vi "grabber stim laser control panel.vi"() -> ()   [LabVIEW 2010]
uses:
  FPGA_ref.ctl
  <vilib>/Platform/TimedLoop/XDataNode/XDataNode.xnode
  <vilib>/Platform/TimedLoop/XDataNode/timing_clust.ctl
  <vilib>/Platform/TimedLoop/XDataNode/nitl_modes.ctl
  <vilib>/Platform/TimedLoop/XDataNode/wakeup.ctl
  <vilib>/rvi/interface/nirviReadWriteControl/nirviReadWriteControl.xnode
  <vilib>/rvi/interface/common/niFpgaNodeNameForErrorReporting.ctl
  <vilib>/rvi/errors/niLvFpgaWhatHappensToTopLevelVI.ctl
  <vilib>/Utility/error.llb/Error Cluster From Error Code.vi
  <vilib>/rvi/errors/niLvFpgaAdjustHostInterfaceError.vi
  <vilib>/Platform/TimedLoop/XDataNode/XDNodeRunTimeDep.lvlib
  NiFpgaLv.dll
panel:
  in  "FPGARef":T1
  in  "laser ref":refnum<vi>
  out "time since last stim":u32
  in  "stop":bool
  in  "auto trig":bool
  in  "stim period (s)":dbl format="%#_3p"
  in  "stim duration (s)":dbl format="%#_3p"
  in  "stim laser on":bool
  # "set to <= 0 for full manual control"
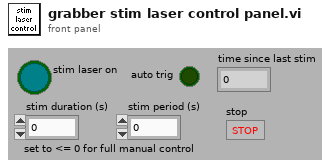
[diagram p1: front panel]
types:
  T1 = typedef "FPGA_ref.ctl" = refnum<k20>
  T2 = typedef "XDNodeRunTimeDep.lvlib/timing_clust.ctl" = cluster{"Expected End [f-1]":u64, "Actual End [f-1]":u64, "Finished Late? [f-1]":bool, "Expected End [i-1]":u64, "Actual End [i-1]":u64, "Finished Late? [i-1]":bool, "Expected Start [i]":u64, "Actual Start [i]":u64, "Expected Start [f]":u64, "Actual Start [f]":u64, "Source Name":string, "Structure Name":string, "Period":i64, "Deadline":i64, "Offset":i64, "Start":i64, "Priority":i32, "Timeout":i32, "Mode":T3, "Wakeup Reason":T4, "Error":errorcluster, "Source Type":string, "Secondary Source Type":string, "Global End Time":u64, "Global Start Time":u64, "Frame Duration":u64, "Iteration Duration":u64, "Assigned CPU":i32, "I/O Scan Engine Mode":u32}
  T3 = typedef "XDNodeRunTimeDep.lvlib/nitl_modes.ctl" = enum32{"No Change", "Process missed periods, maintain original phase", "Discard missed periods, maintain original phase", "Process missed periods, ignore original phase", "Discard missed periods, ignore original phase"}
  T4 = typedef "XDNodeRunTimeDep.lvlib/wakeup.ctl" = enum32{"Normal", "Aborted", "Asynchronous wakeup", "Timing source error", "Timed loop error", "Timeout"}
  T5 = typedef "niFpgaNodeNameForErrorReporting.ctl" = enum16{"Open FPGA VI Reference", "Read/Write Control", "Invoke Method: Abort", "Invoke Method: Acknowledge IRQ", "Invoke Method: Download", "Invoke Method: FIFO.Configure", "Invoke Method: FIFO.Read", "Invoke Method: FIFO.Start", "Invoke Method: FIFO.Stop", "Invoke Method: FIFO.Write", "Invoke Method: Reset", "Invoke Method: Run", "Invoke Method: Wait on IRQ", "Close FPGA VI Reference"}
  T6 = typedef "niLvFpgaWhatHappensToTopLevelVI.ctl" = enum16{"top level VI scripted behind XNode", "top level VI inlined behind XNode"}
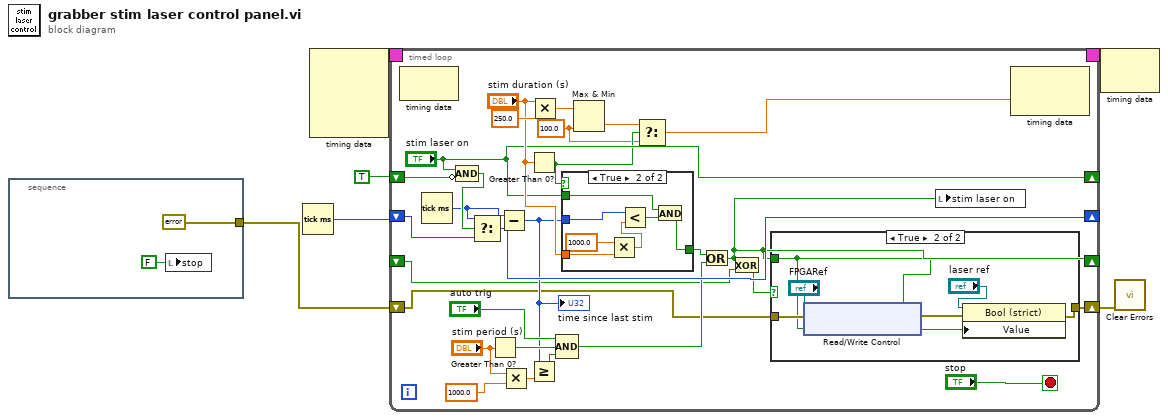
[diagram p0: block diagram]
diagram:
  n1 = stacked-sequence {
    tunnel: [errorcluster {"status"=FALSE, "code"=0, "source"=""} ("error out")] -> w1
    frame #0 {
      n2 = local write "stop"(FALSE ("stop")) -> ()
    }
  }
  n3 = Tick Count (ms)() -> (millisecond timer value=w4:u32)
  n4 = node-c288() -> (w6:T2)  [unwired: 4 in]
  n5 = timed-loop {
    timing: w6 -> [_]
    timing-out: [_] -> w5
    shift-right: ["stim laser on"] -> _
    shift-left: TRUE ("stim laser on") -> [w33]
    shift-right: [w27] -> _
    shift-left: w4 -> [w31]
    shift-right: [w13] -> w2
    shift-left: w1 -> [w12]
    shift-right: [w11] -> _
    shift-left: _ -> [w10]
    stop <- "stop" stop-if-true
    w15 = 100.0 ("y")
    n6 = node-c288() -> ()  [unwired: 1 in, 1 out]
    n7 = Tick Count (ms)() -> (millisecond timer value=w21:u32)
    n8 = Compound Arithmetic op=AND("stim laser on", invert w33) -> (w32:bool)
    n9 = Select(t=w21, s=w32, f=w31) -> (s? t:f=w27:u32)
    n10 = Greater Than 0?(x="stim period (s)") -> (x > 0?=w29:bool)
    n11 = Subtract(x=w21, y=w27) -> (x-y=w23:u32)
    "time since last stim" <- w23
    n12 = Multiply(x="stim period (s)", y=1000.0 ("x")) -> (x*y=w24:dbl)
    n13 = Greater Than 0?(x="stim duration (s)") -> (x > 0?=w17:bool)
    n14 = Greater Or Equal?(x=w23, y=w24) -> (x >= y?=w22:bool)
    n15 = Multiply(x="stim duration (s)", y=250.0) -> (x*y=w34:dbl)
    n16 = Compound Arithmetic op=AND("auto trig", w29, w22) -> (w20:bool)
    n17 = case shown="True" w17 {
      tunnel: "stim duration (s)" -> [_ w90]
      tunnel: [w83 w85] -> w19
      tunnel: "stim laser on" -> [w83 w84]
      tunnel: w23 -> [_ w86]
      frame False {
      }
      frame True {
        n18 = Multiply(x=1000.0, y=w90) -> (x*y=w88:dbl)
        n19 = Less?(x=w86, y=w88) -> (x < y?=w87:bool)
        n20 = And(x=w84, y=w87) -> (x .and. y?=w85:bool)
      }
    }
    n21 = Max & Min(x=w34, y=w15) -> (min(x,y)=w16:dbl)  [unwired: 1 out]
    n22 = Select(t=w16, s=w17, f=w15) -> (s? t:f=w14:dbl)
    n23 = Or(x=w19, y=w20) -> (x .or. y?=w11:bool)
    n24 = Exclusive Or(1:w10, 2:w11) -> (0:w9:bool)
    n25 = case shown="True" w9 {
      tunnel: [w37 w42] -> w13
      tunnel: w12 -> [w37 w41]
      tunnel: w11 -> [_ w39]
      frame False {
      }
      frame True {
        n26 = xnode "Read/Write Control"("FPGA VI Reference In"="FPGARef", "error in"=w41, "stimulus on (low f)"=w39) -> ("error out"=w40:errorcluster)  [unwired: 1 out]
        n27 = property class="Bool (strict)"(reference="laser ref", error in=w40, "Value"=w39) -> (error out=w42:errorcluster)  [unwired: 1 out]
      }
    }
    n28 = local write "stim laser on"(w11) -> ()
    n29 = node-c288(w14) -> ()  [unwired: 1 in, 1 out]
  }
  n30 = node-c288(w5) -> ()  [unwired: 1 out]
  n31 = call <vilib>:"Clear Errors.vi"("error in (no error)"=w2) -> ()  [unwired: 6 in, 1 out]
